vi "robotconstants.vi"() -> ()   [LabVIEW 2020]
panel:
  out "PDH_Current_Channels":cluster{string, dbl}[](array[cluster])=[{"", 0.0}, {"Climber Motor Left", 0.0}, {"Module 3 Azimuth", 0.0}, {"Module 3 Drive", 0.0}, {"Module 2 Azimuth", 0.0}, {"Module 2 Drive", 0.0}, {"Tower Motor", 0.0}, {"Turret Motor", 0.0}, {"Kicker Motor", 0.0}, {"Pneumatics Hub", 0.0}, {"Cowl Motor", 0.0}, {"Shooter Motor Lower", 0.0}, {"Shooter Motor Upper", 0.0}, {"Module 1 Azimuth", 0.0}, {"Module 1 Drive", 0.0}, {"Intake Motor Right", 0.0}, {"Indexer Motor", 0.0}, {"Intake Motor Left", 0.0}, {"Module 0 Drive", 0.0}, {"Module 0 Azimuth", 0.0}, {"Radio Power Module", 0.0}, {"RobotRIO", 0.0}, {"LimeLight", 0.0}, {"LED Spotlights", 0.0}]
  out "Legal_Actuator_Names":string[](array[string])
  out "Legal_Drivers":string[](array[string])
  out "Legal_Auto_Plays":string[](array[string])
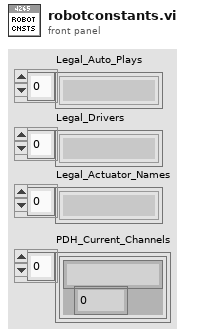
[diagram p1: front panel]
diagram:
